vi "Raw_input_to_sorted.vi"(10 "Input Array":dbl[](array[numeric])) -> (0 "Array data Output":dbl[](array[numeric]), 1 "Array exsist":bool, 3 "Array Out":dbl[](array[numeric]))   [LabVIEW 2016]
doc: "This SubVI takes in Raw Serial Data and sorts it according to its adress"
panel:
  out "date string":string
  out "time string":string
  in  "New array":dbl[](array[numeric])=[0.0, 0.0, 0.0, 0.0, 0.0, 0.0, 0.0, 0.0, 0.0, 0.0, 0.0, 0.0, 0.0, 0.0, 0.0, 0.0, 0.0, 0.0, 0.0, 0.0, 0.0, 0.0, 0.0, 0.0, 0.0, 0.0, 0.0, 0.0, 0.0, 0.0, 0.0, 0.0, 0.0, 0.0, 0.0, 0.0, 0.0, 0.0, 0.0]
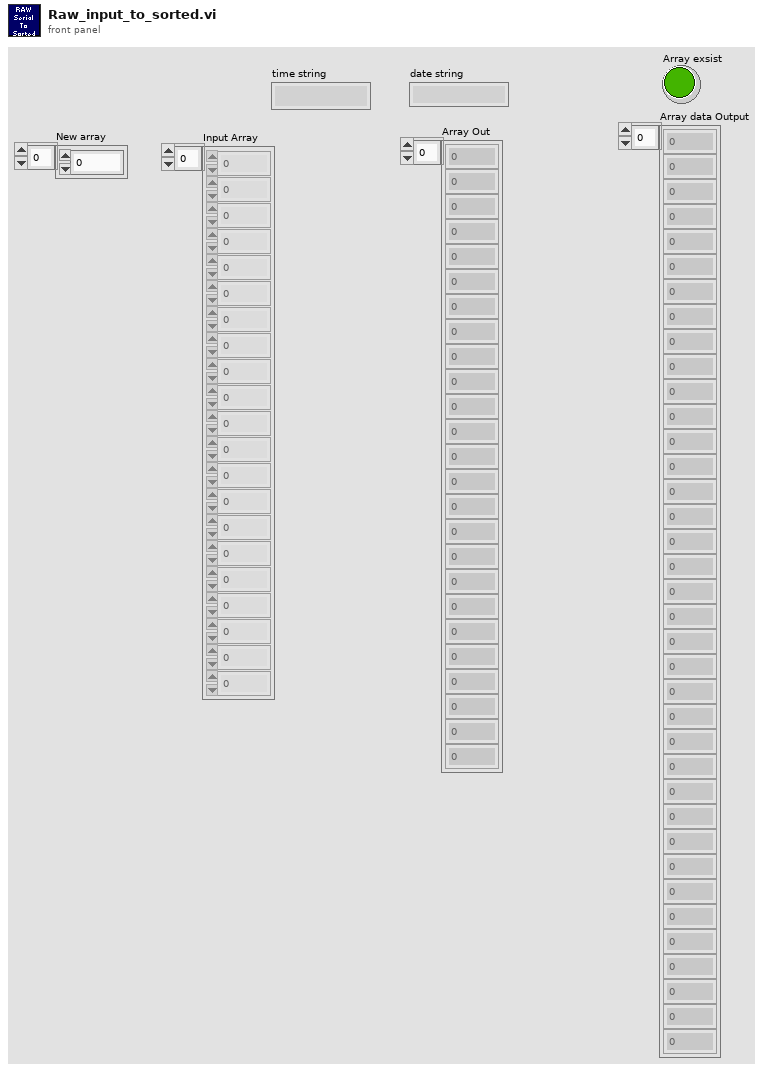
[diagram p1: front panel]
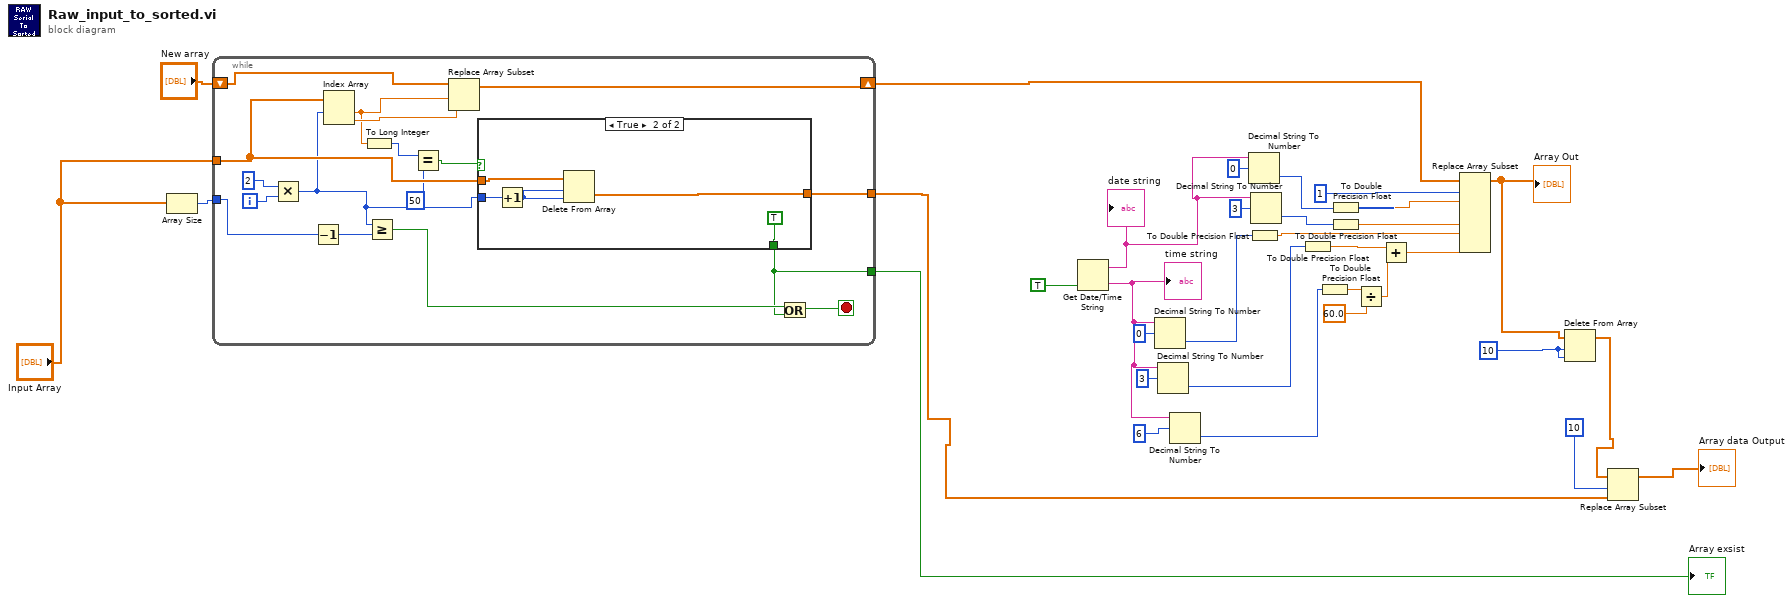
[diagram p0: block diagram]
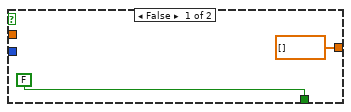
[diagram p2: hidden frame]
diagram:
  w5 = 10 ("length")
  n1 = Array Size(array="Input Array") -> (size(s)=w32:i32)
  n2 = while {
    tunnel: "Input Array" -> [w42]
    tunnel: w32 -> [w47]
    shift-right: [w43] -> w30
    shift-left: "New array" -> [w44]
    tunnel: [w38] -> w2
    tunnel: [w37] -> w11
    i -> [w49]
    stop <- w41 stop-if-true
    n3 = Multiply(x=2, y=w49) -> (x*y=w34:i32)
    n4 = Decrement(x=w47) -> (x-1=w46:i32)
    n5 = Index Array(array=w42, index #1=w34) -> (element #1=w36:dbl, element #2=w50:dbl)  [unwired: 1 in]
    n6 = To Long Integer(number=w36) -> (32bit integer=w35:i32)
    n7 = Greater Or Equal?(x=w34, y=w46) -> (x >= y?=w45:bool)
    n8 = Equal?(x=w35, y=50 ("x")) -> (x = y?=w40:bool)
    n9 = Replace Array Subset(array=w44, new element=w50, index=w36) -> (w43:dbl[])
    n10 = case shown="True" w40 {
      tunnel: w42 -> [_ w57]
      tunnel: w34 -> [_ w55]
      tunnel: [FALSE TRUE] -> w37
      tunnel: [dbl[] [] ("Input Array") w54] -> w38
      frame False {
      }
      frame True {
        n11 = Increment(x=w55) -> (x+1=w53:i32)
        n12 = Delete From Array(array=w57, length=w53, index=w53) -> (deleted portion=w54:dbl[])  [unwired: 1 out]
      }
    }
    n13 = Or(x=w45, y=w37) -> (x .or. y?=w41:bool)
  }
  "Array exsist" <- w11
  n14 = Get Date/Time String(want seconds? (F)=TRUE) -> (date string=w16:string, time string=w26:string)  [unwired: 2 in]
  "time string" <- w26
  "date string" <- w16
  n15 = Decimal String To Number(string=w26, offset=0) -> (number=w23:i32)  [unwired: 1 in, 1 out]
  n16 = Decimal String To Number(string=w26, offset=3) -> (number=w22:i32)  [unwired: 1 in, 1 out]
  n17 = Decimal String To Number(string=w26, offset=6) -> (number=w21:i32)  [unwired: 1 in, 1 out]
  n18 = Decimal String To Number(string=w16, offset=0) -> (number=w12:i32)  [unwired: 1 in, 1 out]
  n19 = To Double Precision Float(number=w23) -> (double precision float=w8:dbl)
  n20 = Decimal String To Number(string=w16, offset=3) -> (number=w13:i32)  [unwired: 1 in, 1 out]
  n21 = To Double Precision Float(number=w22) -> (double precision float=w18:dbl)
  n22 = To Double Precision Float(number=w21) -> (double precision float=w20:dbl)
  n23 = To Double Precision Float(number=w12) -> (double precision float=w10:dbl)
  n24 = To Double Precision Float(number=w13) -> (double precision float=w9:dbl)
  n25 = Divide(x=w20, y=60.0) -> (x/y=w17:dbl)
  n26 = Add(x=w18, y=w17) -> (x+y=w7:dbl)
  n27 = Replace Array Subset(array=w30, new element #1=w10, index #1=1 ("index"), new element #2=w9, new element #3=w8, new element #4=w7) -> (w6:dbl[])  [unwired: 3 in]
  "Array Out" <- w6
  n28 = Delete From Array(array=w6, length=w5, index=w5) -> (array with subset deleted=w4:dbl[])  [unwired: 1 out]
  n29 = Replace Array Subset(array=w4, new element=w2, index=10) -> (→"Array data Output":dbl[])
